vi "InitialisierungDerVariablen.vi"   [LabVIEW 2018]
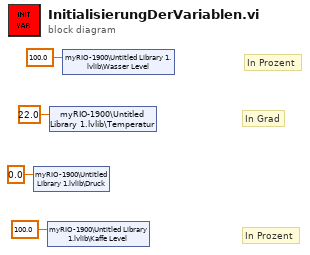
[diagram p0: block diagram]
diagram:
  # "In Prozent"
  # "In Grad"
  # "In Prozent"
  n1 = shared-variable "myRIO-1900\\Untitled Library 1.lvlib\\Druck"(0.0 ("Druck")) -> ()  [unwired: 1 in, 1 out]
  n2 = shared-variable "myRIO-1900\\Untitled Library 1.lvlib\\Kaffe Level"(100.0 ("Kaffe Level")) -> ()  [unwired: 1 in, 1 out]
  n3 = shared-variable "myRIO-1900\\Untitled Library 1.lvlib\\Temperatur"(22.0 ("Temperatur")) -> ()  [unwired: 1 in, 1 out]
  n4 = shared-variable "myRIO-1900\\Untitled Library 1.lvlib\\Wasser Level"(100.0 ("Wasser Level")) -> ()  [unwired: 1 in, 1 out]
